vi "9PalindromeNumber.vi"(8 "error in (no error)":errorcluster, 11 "Numeric":i32) -> (0 "error out":errorcluster, 3 "Boolean":bool)   [LabVIEW 2023]
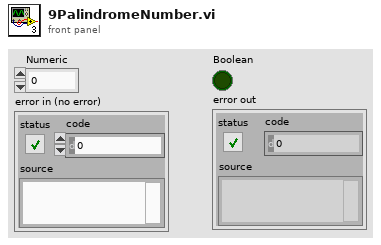
[diagram p1: front panel]
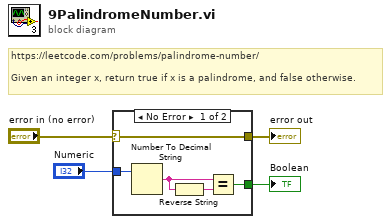
[diagram p0: block diagram]
diagram:
  # "https://leetcode.com/problems/palindrome-number/\n\nGiven an integer x, return true if x is a palindrome, and false otherwise."
  n1 = case shown="No Error" "error in (no error)" {
    selector: "error in (no error)" -> [w9 w10]
    tunnel: [w9 w10] -> w3
    tunnel: [w5 _] -> w2
    tunnel: "Numeric" -> [w8 _]
    frame No Error {
      n2 = Number To Decimal String(number=w8) -> (decimal integer string=w7:string)  [unwired: 1 in]
      n3 = Reverse String(1:w7) -> (0:w6:string)
      n4 = Equal?(x=w7, y=w6) -> (x = y?=w5:bool)
    }
    frame Error {
    }
  }
  "Boolean" <- w2
  "error out" <- w3
